vi "ExSimpleAsync.vi"() -> ()   [LabVIEW 2010]
uses:
  Open-Close/CamHandle.vi
panel:
  in  "Exposure":dbl min=0.0 step=0.001 format="%.3f"
  in  "stop":bool
  in  "Store":bool
  out "error out":errorcluster
  in  "error in (no error)":errorcluster
  # "ExSimipleAsyncExample:\nThis is a Full Frame Async example. This should work with \nall camera systems. It requires a start for every frame \ncollected. Not all timing modes work for all cameras, also \nthe trigger edge only applies to Princeton Instrument \ncameras. Not all cameras have the ability to set the \ntemperature.\nPressing the stop button stops the example."
  # "NOTICE\n\nTHIS VI USES A GLOBAL CAMERA HANDLE\n\nTHE VI EXOPENGLOBALCAM.VI MUST BE\nRUN AT THE START OF THE WORK SESSION.\nTHE CAMERA WILL REMAIN OPENED.\n\nTHE VI EXCLOSEGLOBALCAM.VI MUST\nBE RUN BEFORE LEAVING LABVIEW."
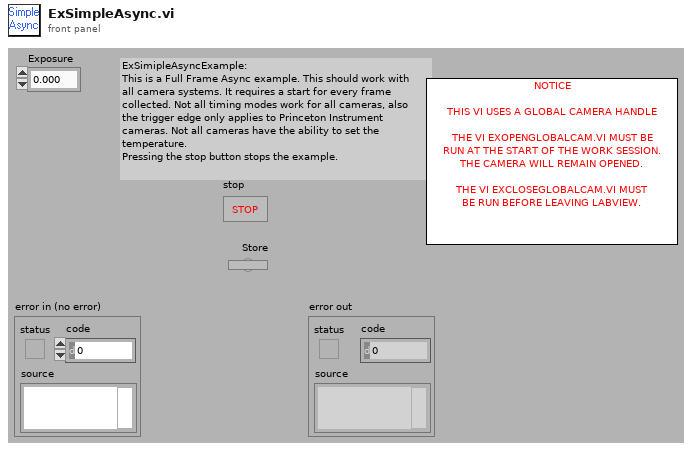
[diagram p1: front panel]
types:
  T1 = cluster{"Acquire mode \n3 is Async":i32, "Exposure":dbl, "Number of Images":i32, "Software Accums":i32}
  T2 = cluster{"Camera Handle":u32, "File Handle":u32, "Display Handle":u32, "Image Handle":u32}
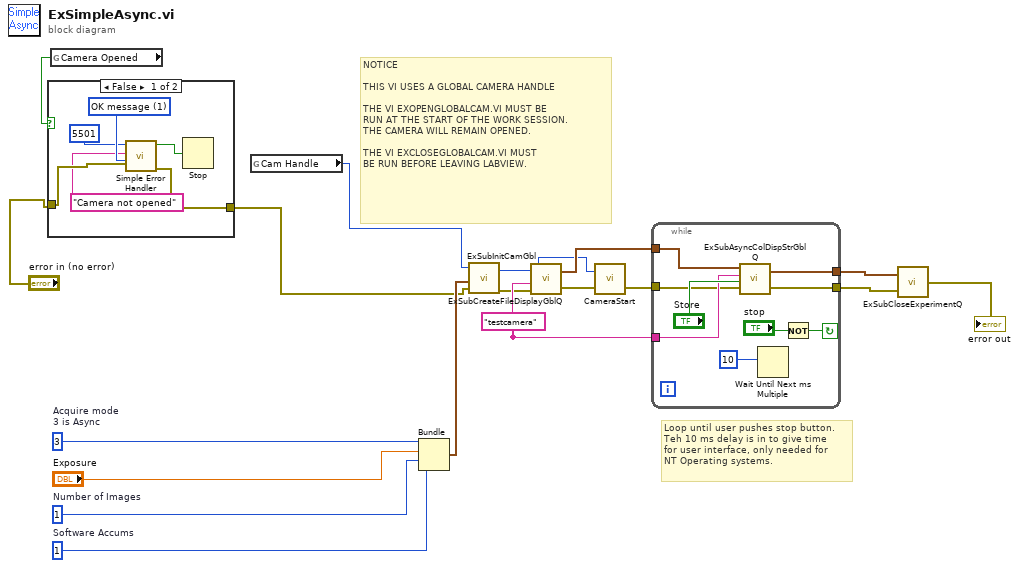
[diagram p0: block diagram]
diagram:
  w16 = 1  # Number of Images
  w17 = 3  # Acquire mode  3 is Async
  w15 = 1  # Software Accums
  w18 = "testcamera"
  # "NOTICE\n\nTHIS VI USES A GLOBAL CAMERA HANDLE\n\nTHE VI EXOPENGLOBALCAM.VI MUST BE\nRUN AT THE START OF THE WORK SESSION.\nTHE CAMERA WILL REMAIN OPENED.\n\nTHE VI EXCLOSEGLOBALCAM.VI MUST\nBE RUN BEFORE LEAVING LABVIEW."
  # "Loop until user pushes stop button.\nTeh 10 ms delay is in to give time \nfor user interface, only needed for \nNT Operating systems."
  n1 = global read "CamHandle.vi" "Camera Opened"() -> (w6:bool)
  n2 = case shown="False" w6 {
    tunnel: "error in (no error)" -> [w23 w25]
    tunnel: [w22 w25] -> w2
    frame False {
      w24 = u16 1 items=["no dialog", "OK message", "continue or stop message"] ("type of dialog (OK msg:1)")
      n3 = call <vilib>:"Simple Error Handler.vi"("error code (no error:0)"=5501, "error source (\" \")"="Camera not opened", "type of dialog (OK msg:1)"=w24, "error in (no error)"=w23) -> ("error?"=w20:bool, "error out"=w22:errorcluster)  [unwired: 1 in, 3 out]
      n4 = Stop(stop? (T)=w20) -> ()
    }
    frame True {
    }
  }
  n5 = global read "CamHandle.vi" "Cam Handle"() -> (w1:u32)
  n6 = Bundle("Acquire mode \n3 is Async"=w17, "Exposure"="Exposure", "Number of Images"=w16, "Software Accums"=w15) -> (w13:T1)  [unwired: 1 in]
  n7 = call "ExSubInitCamGbl.vi"("error in (no error)"=w2, "Camera Information"=w13, "Camera Handle"=w1) -> ("error out"=w12:errorcluster, "Camera Handle"=w8:u32)
  n8 = call "ExSubCreateFileDisplayGblQ.vi"("error in (no error)"=w12, "File and Display Name"=w18, "Camera Handle"=w8) -> ("error out"=w11:errorcluster, "Handles Out"=w10:T2)  [unwired: 1 in]
  n9 = call <userlib>:"CameraStart.vi"("error in"=w11, "Camera Handle"=w8) -> ("error out"=w9:errorcluster)  [unwired: 1 out]
  n10 = while {
    tunnel: w10 -> [w26]
    tunnel: w9 -> [w31]
    tunnel: w18 -> [w32]
    tunnel: [w29] -> w4
    tunnel: [w30] -> w5
    stop <- w28 continue-if-true
    n11 = call "ExSubAsyncColDispStrGblQ.vi"("error in (no error)"=w31, "Store Data"="Store", "Display Title"=w32, "Handle Cluster"=w26) -> ("error out"=w29:errorcluster, "Handle Cluster Out"=w30:T2)
    n12 = Wait Until Next ms Multiple(millisecond multiple=10) -> ()  [unwired: 1 out]
    n13 = Not(x="stop") -> (.not. x?=w28:bool)
  }
  n14 = call "ExSubCloseExperimentQ.vi"("error in (no error)"=w4, "Handles In"=w5) -> ("error out"=→"error out":errorcluster)
